vi "Launcher.vi"() -> ()   [LabVIEW 2018]
uses:
  Host-DQMH/Main-Module/Host Main.lvlib
panel:
  out "error out":errorcluster
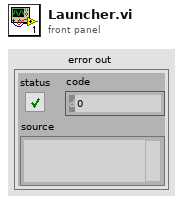
[diagram p1: front panel]
types:
  T1 = enum32{"Invalid", "Standard", "Closed", "Hidden", "Minimized", "Maximized"}
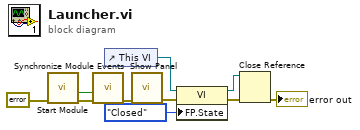
[diagram p0: block diagram]
diagram:
  n1 = call "Start Module.vi"("error in"=errorcluster {"status"=FALSE, "code"=0, "source"=""}) -> ("error out"=w4:errorcluster, "Wait for Event Sync?"=w3:bool)  [unwired: 7 in, 2 out]
  n2 = call "Synchronize Module Events.vi"("error in"=w4, "Wait for Event Sync?"=w3) -> ("error out"=w2:errorcluster)  [unwired: 9 in]
  n3 = control-ref of="This VI"() -> (w10:refnum<vi>)
  n4 = call "Show Panel.vi"("error in"=w2) -> ("error out"=w1:errorcluster)  [unwired: 10 in]
  n5 = property class="VI"(reference=w10, error in=w1, "FP.State"=T1."Closed" ("Front Panel Window:State")) -> (reference out=w7:refnum<vi>, error out=w8:errorcluster)
  n6 = Close Reference(reference=w7, error in (no error)=w8) -> (error out=→"error out":errorcluster)
